vi "File System Query.vi"(8 "error in (no error)":errorcluster, 11 "VISA resource name":refnum<visa-resource-name>) -> (0 "error out":errorcluster, 1 "Folder Names":string[](array[string]), 2 "Filenames":string[](array[string]), 3 "VISA resource name out":refnum<visa-resource-name>, 4 "Free Space (Byte)":dbl, 5 "Current Working Directory":string)   [LabVIEW 2009, in "Tektronix DPO MSO 2000 4000 Series.lvlib"]
doc: "Queries the oscilloscope for file system commands."
uses:
  <instrlib>/Tektronix DPO MSO 2000 4000 Series/Tektronix DPO MSO 2000 4000 Series.lvlib
  <vilib>/regexp/Match Regular Expression.xnode
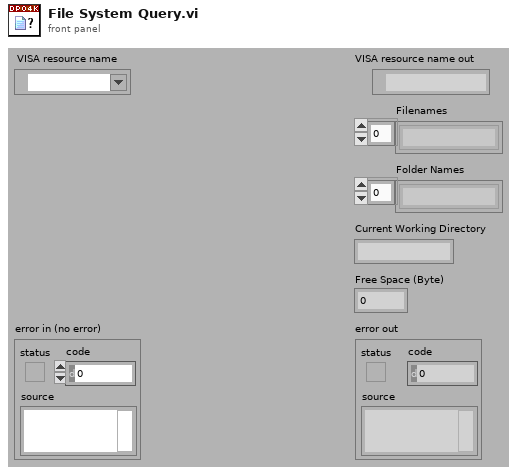
[diagram p1: front panel]
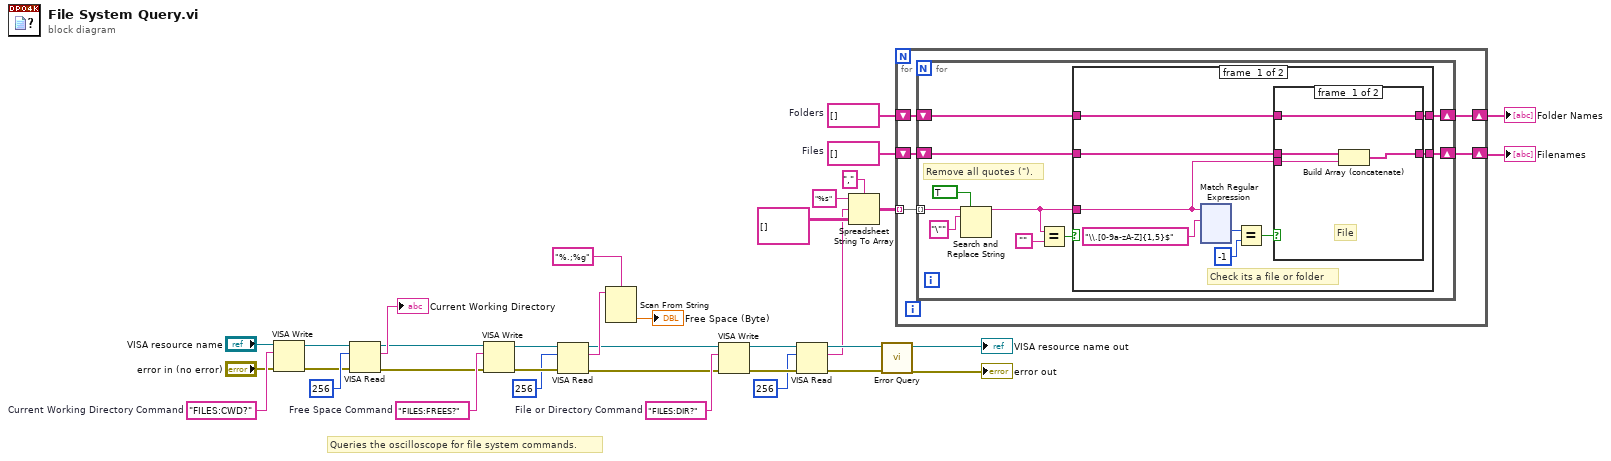
[diagram p0: block diagram]
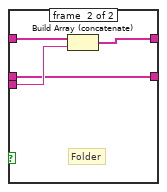
[diagram p2: hidden frame]
diagram:
  w15 = string[] []  # Files
  w14 = string[] []  # Folders
  w24 = "FILES:FREES?"  # Free Space Command
  w26 = "FILES:CWD?"  # Current Working Directory Command
  w35 = "FILES:DIR?"  # File or Directory Command
  # "Queries the oscilloscope for file system commands."
  n1 = VISA Write(VISA resource name="VISA resource name", write buffer=w26, error in (no error)="error in (no error)") -> (VISA resource name out=w27:refnum<visa-resource-name>, error out=w28:errorcluster)  [unwired: 1 out]
  n2 = VISA Read(VISA resource name=w27, byte count=u32 256, error in (no error)=w28) -> (VISA resource name out=w19:refnum<visa-resource-name>, read buffer=→"Current Working Directory":string, error out=w20:errorcluster)  [unwired: 1 out]
  n3 = VISA Write(VISA resource name=w19, write buffer=w24, error in (no error)=w20) -> (VISA resource name out=w23:refnum<visa-resource-name>, error out=w22:errorcluster)  [unwired: 1 out]
  n4 = VISA Read(VISA resource name=w23, byte count=u32 256, error in (no error)=w22) -> (VISA resource name out=w7:refnum<visa-resource-name>, read buffer=w18:string, error out=w5:errorcluster)  [unwired: 1 out]
  n5 = Scan From String(format string="%.;%g", input string=w18) -> (output 1=→"Free Space (Byte)":dbl)  [unwired: 3 in, 3 out]
  n6 = VISA Write(VISA resource name=w7, write buffer=w35, error in (no error)=w5) -> (VISA resource name out=w32:refnum<visa-resource-name>, error out=w31:errorcluster)  [unwired: 1 out]
  n7 = VISA Read(VISA resource name=w32, byte count=u32 256, error in (no error)=w31) -> (VISA resource name out=w6:refnum<visa-resource-name>, read buffer=w3:string, error out=w4:errorcluster)  [unwired: 1 out]
  n8 = Spreadsheet String To Array(delimiter (Tab)=",", format string="%s", spreadsheet string=w3, array type (2D Dbl)=string[][] [] ("array")) -> (array=w13:string[][])
  n9 = call <instrlib>:"Error Query.vi"("error in (no error)"=w4, "VISA resource name"=w6) -> ("error out"=→"error out":errorcluster, "VISA resource name out"=→"VISA resource name out":refnum<visa-resource-name>)  [unwired: 6 in, 2 out]
  n10 = for {
    tunnel: w13 -> [w40] mode=indexing
    shift-right: [w38] -> w2
    shift-left: w14 -> [w39]
    shift-right: [w36] -> w1
    shift-left: w15 -> [w37]
    n11 = for {
      tunnel: w40 -> [w48] mode=indexing
      shift-right: [w46] -> w38
      shift-left: w39 -> [w47]
      shift-right: [w44] -> w36
      shift-left: w37 -> [w45]
      # "Remove all quotes (\")."
      n12 = Search and Replace String(replace all?=TRUE ("replace all? (F)"), input string=w48, search string="\"") -> (result string=w42:string)  [unwired: 5 in, 3 out]
      n13 = Equal?(x=w42, y="") -> (x = y?=w41:bool)
      n14 = case shown="False" w41 {
        tunnel: w47 -> [w55 w176]
        tunnel: [w54 w176] -> w46
        tunnel: w45 -> [w53 w175]
        tunnel: [w52 w175] -> w44
        tunnel: w42 -> [w51 _]
        frame #0 {
          # "Check its a file or folder"
          n15 = xnode "Match Regular Expression"("input string"=w51, "regular expression"="\\.[0-9a-zA-Z]{1,5}$") -> ("offset past match"=w58:i32)  [unwired: 4 in, 4 out]
          n16 = Equal?(x=w58, y=-1) -> (x = y?=w56:bool)
          n17 = case shown="True" w56 {
            tunnel: w55 -> [w63 w67]
            tunnel: w51 -> [w60 w66]
            tunnel: [w63 w65] -> w54
            tunnel: w53 -> [w62 w64]
            tunnel: [w61 w64] -> w52
            frame #0 {
              # "File"
              n18 = Build Array (concatenate)(w62, w60) -> (w61:string[])
            }
            frame #1 {
              # "Folder"
              n19 = Build Array (concatenate)(w67, w66) -> (w65:string[])
            }
          }
        }
        frame #1 {
        }
      }
    }
  }
  "Filenames" <- w1
  "Folder Names" <- w2
